vi "Feedback Factorial.vi"() -> ()   [LabVIEW 2020]
panel:
  in  "Numeric 2":i32
  out "Factorial":i32
  # "Feedback Factorial"
  # "1x1 =1\n2x1 =2\n2x3 =6\n6x4 =24\n24x5 =125"
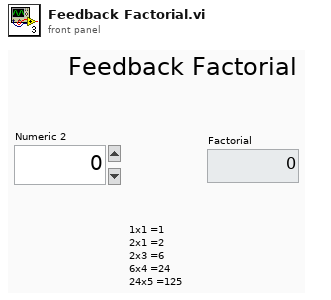
[diagram p1: front panel]
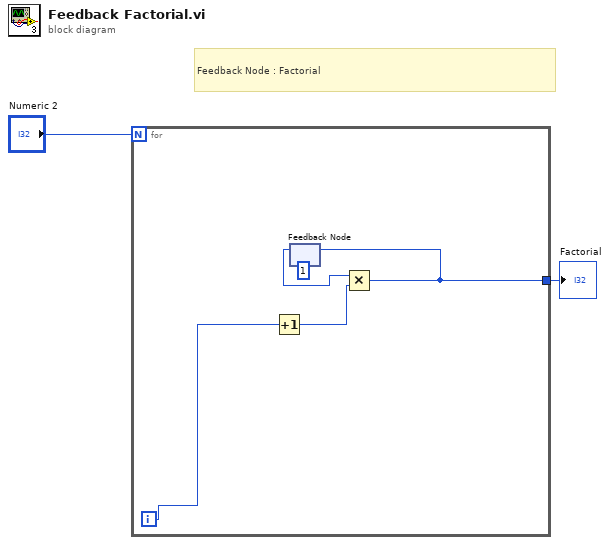
[diagram p0: block diagram]
diagram:
  # "Feedback Node : Factorial"
  n1 = for {
    N: "Numeric 2" -> [_]
    tunnel: [w3] -> w2
    i -> [w6]
    n2 = Increment(x=w6) -> (x+1=w7:i32)
    n3 = feedback #1(1) -> (w5:i32)
    n4 = Multiply(x=w5, y=w7) -> (x*y=w3:i32)
    n5 = feedback-in #1(w3) -> ()
  }
  "Factorial" <- w2
